vi "Vision Tracking Drive Control.vi"(11 "Cluster In":T11) -> (3 "Cluster Out":T11)   [LabVIEW 2018]
uses:
  <vilib>/Rock Robotics/WPI/MotorControl/WPI_MotorControlDeviceRef.ctl
  <vilib>/Rock Robotics/WPI/MotorControl/WPI_MotorControlType.ctl
  <vilib>/Rock Robotics/SystemInterfaces/DIO/FPGA_DIOPWMChannel.ctl
  <vilib>/Rock Robotics/WPI/PWM/WPI_PWMDeadband.ctl
  <vilib>/Rock Robotics/SystemInterfaces/DIO/FPGA_DIOChannel.ctl
  <vilib>/Rock Robotics/WPI/Joystick/WPI_JoystickDevRef.ctl
  <vilib>/Rock Robotics/WPI/Joystick/WPI_JoystickDeviceEnum.ctl
  <vilib>/Rock Robotics/WPI/DriverStation/WPI_DriverStationRobotMode2.ctl
  <vilib>/Rock Robotics/WPI/RobotDrive/WPI_RobotDriveDevRef.ctl
  Vision States.ctl
  <vilib>/Rock Robotics/WPI/ThirdParty/Phoenix-LabVIEW/Motor Controller/Controls/CTRE_Phoenix_MotorControl_ControlMode.ctl
  <vilib>/Rock Robotics/Network Tables/NT Read Number.vi
  Robot Global Data.vi
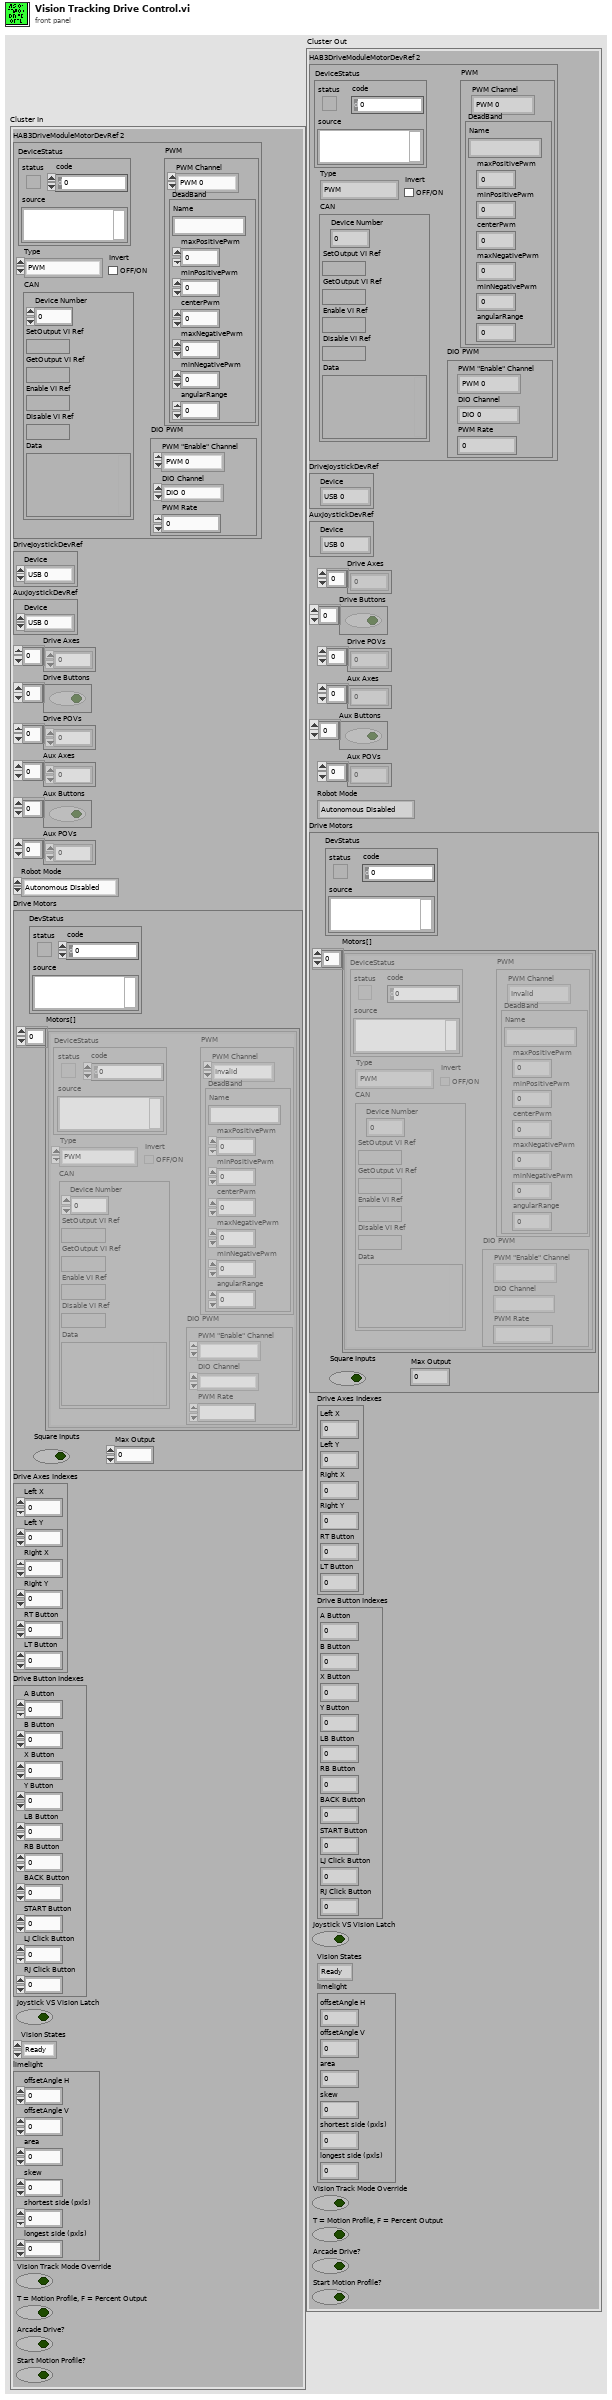
[diagram p1: front panel]
types:
  T1 = typedef "WPI_MotorControlDeviceRef.ctl" = cluster{"DeviceStatus":errorcluster, "Type":T2, "PWM":cluster{"PWM Channel":T3, "DeadBand":T4}, "CAN":cluster{"Device Number":u8, "SetOutput VI Ref":variant, "GetOutput VI Ref":variant, "Enable VI Ref":variant, "Disable VI Ref":variant, "Data":variant}, "Invert":bool, "DIO PWM":cluster{"PWM \"Enable\" Channel":T3, "DIOChannel":T5, "PWM Rate":dbl}}
  T2 = typedef "WPI_MotorControlType.ctl" = enum16{"PWM", "CAN", "DIO PWM"}
  T3 = typedef "FPGA_DIOPWMChannel.ctl" = enum8{"PWM 0", "PWM 1", "PWM 2", "PWM 3", "PWM 4", "PWM 5", "PWM 6", "PWM 7", "PWM 8", "PWM 9", "PWM MXP 0", "PWM MXP 1", "PWM MXP 2", "PWM MXP 3", "PWM MXP 4", "PWM MXP 5", "PWM MXP 6", "PWM MXP 7", "PWM MXP 8", "PWM MXP 9", "Invalid"}
  T4 = typedef "WPI_PWMDeadband.ctl" = cluster{"Name":string, "maxPositivePwm":i32, "minPositivePwm":i32, "centerPwm":i32, "maxNegativePwm":i32, "minNegativePwm":i32, "angularRange":u16}
  T5 = typedef "FPGA_DIOChannel.ctl" = enum8{"DIO 0", "DIO 1", "DIO 2", "DIO 3", "DIO 4", "DIO 5", "DIO 6", "DIO 7", "DIO 8", "DIO 9", "DIO MXP 0", "DIO MXP 1", "DIO MXP 2", "DIO MXP 3", "DIO MXP 4", "DIO MXP 5", "DIO MXP 6", "DIO MXP 7", "DIO MXP 8", "DIO MXP 9", "DIO MXP 10", "DIO MXP 11", "DIO MXP 12", "DIO MXP 13", "DIO MXP 14", "DIO MXP 15", "SPI Port CS1", "SPI Port CS2", "SPI Port CS3", "SPI Port MISO", "SPI Port MOSI", "Invalid"}
  T6 = typedef "WPI_JoystickDevRef.ctl" = cluster{"Device":T7}
  T7 = typedef "WPI_JoystickDeviceEnum.ctl" = enum16{"USB 0", "USB 1", "USB 2", "USB 3", "USB 4", "USB 5"}
  T8 = typedef "WPI_DriverStationRobotMode2.ctl" = enum16{"Autonomous Disabled", "Autonomous Enabled", "Teleop Disabled", "Teleop Enabled", "Disconnected", "Finish", "Test Disabled", "Test Enabled", "Emergency Stopped"}
  T9 = typedef "WPI_RobotDriveDevRef.ctl" = cluster{"DevStatus":errorcluster, "Motors[]":T1[], "Square Inputs":bool, "Max Output":dbl}
  T10 = typedef "Vision States.ctl" = enum16{"Ready", "Forward Until Target at Edge", "Vision Track"}
  T11 = cluster{"HAB3DriveModuleMotorDevRef 2":T1, "DriveJoystickDevRef":T6, "AuxJoystickDevRef":T6, "Drive Axes":dbl[], "Drive Buttons":bool[], "Drive POVs":i16[], "Aux Axes":dbl[], "Aux Buttons":bool[], "Aux POVs":i16[], "Robot Mode":T8, "Drive Motors":T9, "Drive Axes Indexes":cluster{"Left X":i32, "Left Y":i32, "Right X":i32, "Right Y":i32, "RT Button":i32, "LT Button":i32}, "Drive Button Indexes":cluster{"A Button":i32, "B Button":i32, "X Button":i32, "Y Button":i32, "LB Button":i32, "RB Button":i32, "BACK Button":i32, "START Button":i32, "LJ Click Button":i32, "RJ Click Button":i32}, "Joystick VS Vision Latch":bool, "Vision States":T10, "limelight":cluster{"offsetAngle H":dbl, "offsetAngle V":dbl, "area":dbl, "skew":dbl, "shortest side (pxls)":dbl, "longest side (pxls)":dbl}, "Vision Track Mode Override":bool, "T = Motion Profile, F = Percent Output":bool, "Arcade Drive?":bool, "Start Motion Profile?":bool}
  T12 = typedef "Which Robot Enum.ctl" = enum16{"Competition Bot", "Practice Bot", "Code Bot"}
  T13 = typedef "CTRE_Phoenix_MotorControl_ControlMode.ctl" = u16
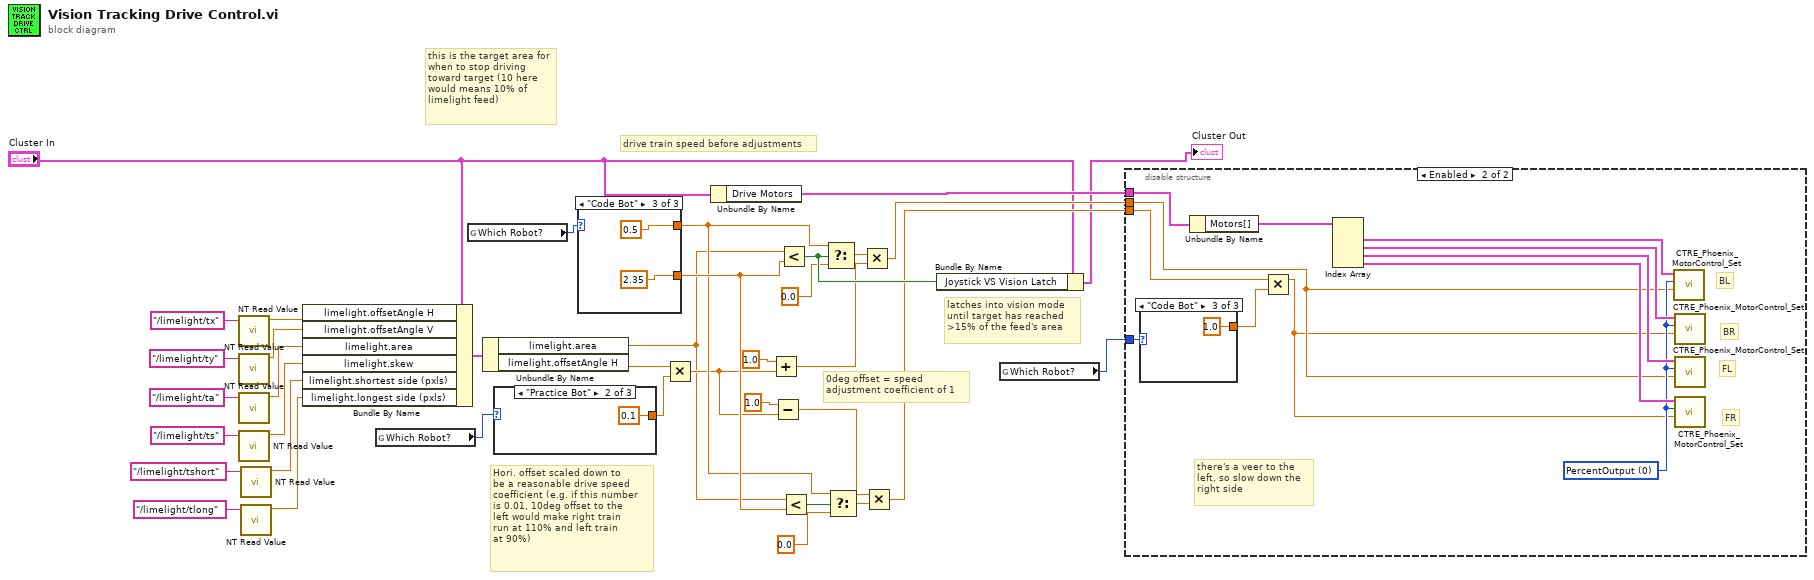
[diagram p0: block diagram]
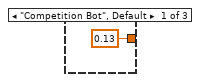
[diagram p2: hidden frame]
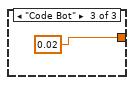
[diagram p3: hidden frame]
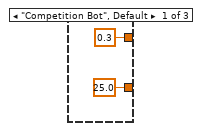
[diagram p4: hidden frame]
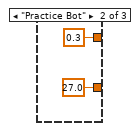
[diagram p5: hidden frame]
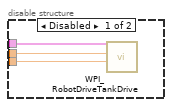
[diagram p6: hidden frame]
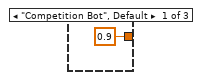
[diagram p7: hidden frame]
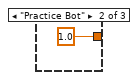
[diagram p8: hidden frame]
diagram:
  # "latches into vision mode \nuntil target has reached \n>15% of the feed's area"
  # "drive train speed before adjustments"
  # "this is the target area for\nwhen to stop driving \ntoward target (10 here \nwould means 10% of \nlimelight feed)"
  # "Hori. offset scaled down to\nbe a reasonable drive speed\ncoefficient (e.g. if this number\nis 0.01, 10deg offset to the \nleft would make right train \nrun at 110% and left train \nat 90%)"
  # "0deg offset = speed \nadjustment coefficient of 1"
  n1 = call-poly <vilib>:"NT Read Value.vi"("Name"="/limelight/tx") -> ("Numeric"=w10:dbl)  [unwired: 9 in, 1 out]
  n2 = call-poly <vilib>:"NT Read Value.vi"("Name"="/limelight/ty") -> ("Numeric"=w11:dbl)  [unwired: 9 in, 1 out]
  n3 = call-poly <vilib>:"NT Read Value.vi"("Name"="/limelight/ta") -> ("Numeric"=w12:dbl)  [unwired: 9 in, 1 out]
  n4 = call-poly <vilib>:"NT Read Value.vi"("Name"="/limelight/ts") -> ("Numeric"=w13:dbl)  [unwired: 9 in, 1 out]
  n5 = call-poly <vilib>:"NT Read Value.vi"("Name"="/limelight/tshort") -> ("Numeric"=w36:dbl)  [unwired: 9 in, 1 out]
  n6 = call-poly <vilib>:"NT Read Value.vi"("Name"="/limelight/tlong") -> ("Numeric"=w37:dbl)  [unwired: 9 in, 1 out]
  n7 = Bundle By Name(cluster="Cluster In", "limelight.offsetAngle H"=w10, "limelight.offsetAngle V"=w11, "limelight.area"=w12, "limelight.skew"=w13, "limelight.shortest side (pxls)"=w36, "limelight.longest side (pxls)"=w37) -> (w14:T11)
  n8 = global read "Robot Global Data.vi" "Which Robot?"() -> (w4:T12)
  n9 = global read "Robot Global Data.vi" "Which Robot?"() -> (w5:T12)
  n10 = Unbundle By Name(w14) -> ("limelight.area"=w25:dbl, "limelight.offsetAngle H"=w17:dbl)
  n11 = case shown="\"Practice Bot\"" w4 {
    tunnel: [0.13 ("y") 0.1 ("y") 0.02 ("y")] -> w18
    frame "Competition Bot", Default {
    }
    frame "Practice Bot" {
    }
    frame "Code Bot" {
    }
  }
  n12 = case shown="\"Code Bot\"" w5 {
    tunnel: [25.0 27.0 2.35] -> w31
    tunnel: [0.3 ("t") 0.3 ("t") 0.5 ("t")] -> w30
    frame "Competition Bot", Default {
    }
    frame "Practice Bot" {
    }
    frame "Code Bot" {
    }
  }
  n13 = Multiply(x=w17, y=w18) -> (x*y=w28:dbl)
  n14 = Unbundle By Name("Cluster In") -> ("Drive Motors"=w32:T9)
  n15 = Add(x=1.0, y=w28) -> (x+y=w22:dbl)
  n16 = Subtract(x=1.0, y=w28) -> (x-y=w29:dbl)
  n17 = Less?(x=w25, y=w31) -> (x < y?=w33:bool)
  n18 = Less?(x=w25, y=w31) -> (x < y?=w21:bool)
  n19 = Select(t=w30, s=w33, f=0.0) -> (s? t:f=w16:dbl)
  n20 = Select(t=w30, s=w21, f=0.0) -> (s? t:f=w24:dbl)
  n21 = Multiply(x=w16, y=w22) -> (x*y=w19:dbl)
  n22 = Multiply(x=w29, y=w24) -> (x*y=w26:dbl)
  n23 = Bundle By Name(cluster="Cluster In", "Joystick VS Vision Latch"=w33) -> (→"Cluster Out":T11)
  n24 = global read "Robot Global Data.vi" "Which Robot?"() -> (w3:T12)
  n25 = disable-structure shown="Enabled" {
    disable-tunnel: w32 -> [w49 w55]
    disable-tunnel: w26 -> [w48 w53]
    disable-tunnel: w19 -> [w47 w54]
    disable-tunnel: w3 -> [_ w50]
    frame Disabled {
      n26 = call <vilib>:"WPI_RobotDriveTankDrive.vi"("Right axis value"=w48, "Left axis value"=w47, "RobotDriveDevRef"=w49) -> ()  [unwired: 6 in, 3 out]
    }
    frame Enabled {
      w56 = T13 0 items=["PercentOutput"=0, "Position"=1, "Velocity"=2, "Current"=3, "Follower"=5, "MotionProfile"=6, "MotionMagic"=7, "MotionProfileArc"=10, "Disabled"=15] ("Control Mode")
      # "there's a veer to the\nleft, so slow down the\nright side"
      # "FR"
      # "FL"
      # "BR"
      # "BL"
      n27 = case shown="\"Code Bot\"" w50 {
        tunnel: [0.9 ("y") 1.0 ("y") 1.0 ("y")] -> w51
        frame "Competition Bot", Default {
        }
        frame "Practice Bot" {
        }
        frame "Code Bot" {
        }
      }
      n28 = Unbundle By Name(w55) -> ("Motors[]"=w61:T1[])
      n29 = Multiply(x=w53, y=w51) -> (x*y=w52:dbl)
      n30 = Index Array(array=w61) -> (element #1=w60:T1, element #2=w57:T1, element #3=w59:T1, element #4=w58:T1)  [unwired: 4 in]
      n31 = call <vilib>:"CTRE_Phoenix_MotorControl_Set.vi"("Output"=w54, "Control Mode"=w56, "PhoenixMotorControlDevRef"=w60) -> ()  [unwired: 7 in, 2 out]
      n32 = call <vilib>:"CTRE_Phoenix_MotorControl_Set.vi"("Output"=w52, "Control Mode"=w56, "PhoenixMotorControlDevRef"=w57) -> ()  [unwired: 7 in, 2 out]
      n33 = call <vilib>:"CTRE_Phoenix_MotorControl_Set.vi"("Output"=w54, "Control Mode"=w56, "PhoenixMotorControlDevRef"=w59) -> ()  [unwired: 7 in, 2 out]
      n34 = call <vilib>:"CTRE_Phoenix_MotorControl_Set.vi"("Output"=w52, "Control Mode"=w56, "PhoenixMotorControlDevRef"=w58) -> ()  [unwired: 7 in, 2 out]
    }
  }
